vi "Destroy.vi"(8 "error in (no error)":errorcluster, 11 "TreeNodeArray in":refnum<class "TreeNodeArray.lvclass">) -> (0 "error out":errorcluster)   [LabVIEW 2013, in "MDSplus.lvlib" / "TreeNodeArray.lvclass"]
uses:
  <vilib>/MDSplus/Classes/TreeNodeArray_Class/TreeNodeArray.lvclass
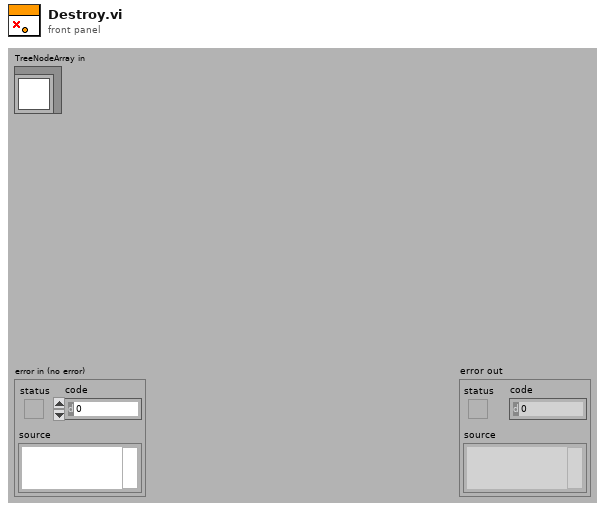
[diagram p1: front panel]
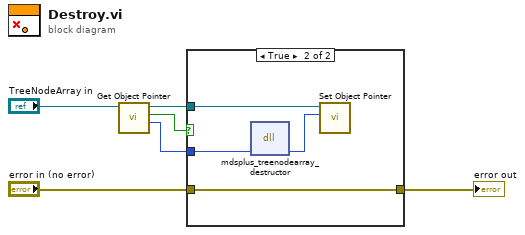
[diagram p0: block diagram]
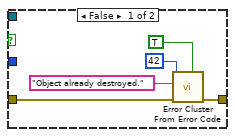
[diagram p2: hidden frame]
diagram:
  n1 = call-dynamic "Get Object Pointer.vi"("TreeNodeArray in"="TreeNodeArray in") -> ("Object Pointer"=w3:i64, "Assigned object pointer?"=w4:bool, "TreeNodeArray out"=w6:refnum<class "TreeNodeArray.lvclass">)  [unwired: 8 in]
  n2 = case shown="True" w4 {
    tunnel: w6 -> [_ w15]
    tunnel: w3 -> [_ w14]
    tunnel: "error in (no error)" -> [w11 w12]
    tunnel: [w8 w12] -> w1
    frame False {
      n3 = call <vilib>:"Error Cluster From Error Code.vi"("is warning? (False)"=TRUE, "error in (no error)"=w11, "error message (\"\")"="Object already destroyed." ("error message (\"\")"), "error code (0)"=42) -> ("error out"=w8:errorcluster)  [unwired: 5 in]
    }
    frame True {
      n4 = dll-call lib="MDSobjectsLVShr" fn="mdsplus_treenodearray_destructor"("lvTreeNodeArrayPtr"=w14) -> ("lvTreeNodeArrayPtr"=w13:i64)  [unwired: 4 in, 2 out]
      n5 = call-dynamic "Set Object Pointer.vi"("Object Pointer"=w13, "TreeNodeArray in"=w15) -> ()  [unwired: 9 in, 1 out]
    }
  }
  "error out" <- w1
